vi "latchBool.vi"(1 "Trigger Edge":enum16{"Falling Edge", "Rising Edge"}(ring)=enum."Rising Edge", 2 "in":bool) -> (0 "out":bool)   [LabVIEW 2012]
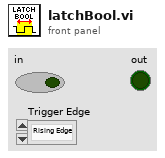
[diagram p1: front panel]
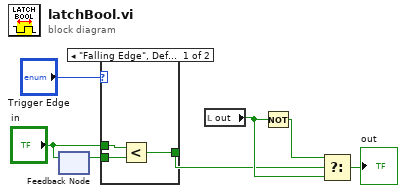
[diagram p0: block diagram]
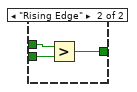
[diagram p2: hidden frame]
diagram:
  n1 = feedback-in #1("in") -> ()
  n2 = feedback #1() -> (w7:bool)  [unwired: 1 in]
  n3 = case shown="\"Falling Edge\", Default" "Trigger Edge" {
    tunnel: w7 -> [w10 w13]
    tunnel: "in" -> [w9 w12]
    tunnel: [w8 w11] -> w1
    frame "Falling Edge", Default {
      n4 = Less?(x=w9, y=w10) -> (x < y?=w8:bool)
    }
    frame "Rising Edge" {
      n5 = Greater?(x=w12, y=w13) -> (0:w11:bool)
    }
  }
  n6 = local read "out"() -> (w2:bool)
  n7 = Not(x=w2) -> (.not. x?=w3:bool)
  n8 = Select(t=w3, s=w1, f=w2) -> (s? t:f=→"out":bool)
